vi "Double HWSync.vi"() -> ()   [LabVIEW 2014]
doc: "Use this template to build a producer/consumer design pattern with events to produce queue items. Use this design pattern instead of the User Interface Event Handler pattern for user interfaces when you want to execute code asynchronously in response to an event without slowing the user interface responsiveness."
uses:
  APIs/Message Queue/Enqueue Message (Single).vi
  APIs/Message Queue/Enqueue Message (Array).vi
  HWSyncLoop/HWSyncLoop.lvlib
  APIs/Message Queue/WINFAS 2 Message Queue.lvlib
panel:
  in  "SEND":bool
  in  "LOAD DRIVER":bool
  in  "Ruta a Driver":path=path "D:/Repositorio MAGNIS/INF002/v0/Modules/HAL/DriverMasterSync/build/DriverMasterSync.lvlibp"
  in  "Mensaje":string
  in  "stop":bool
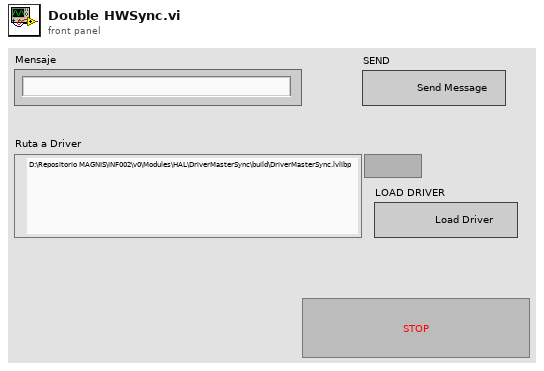
[diagram p1: front panel]
types:
  T1 = typedef "WINFAS 2 Message Queue.lvlib/All Message Queues.ctl" = cluster{"CORE":refnum<queue>, "HAL":refnum<queue>, "HWSync1":refnum<queue>, "HWSync2":refnum<queue>, "HWSync3":refnum<queue>, "HWSync4":refnum<queue>, "HWSync5":refnum<queue>, "HWAsync":refnum<queue>, "Event UI":refnum<queue>, "Display UI":refnum<queue>, "MATH":refnum<queue>, "SEQ":refnum<queue>, "DB":refnum<queue>, "ERR":refnum<queue>}
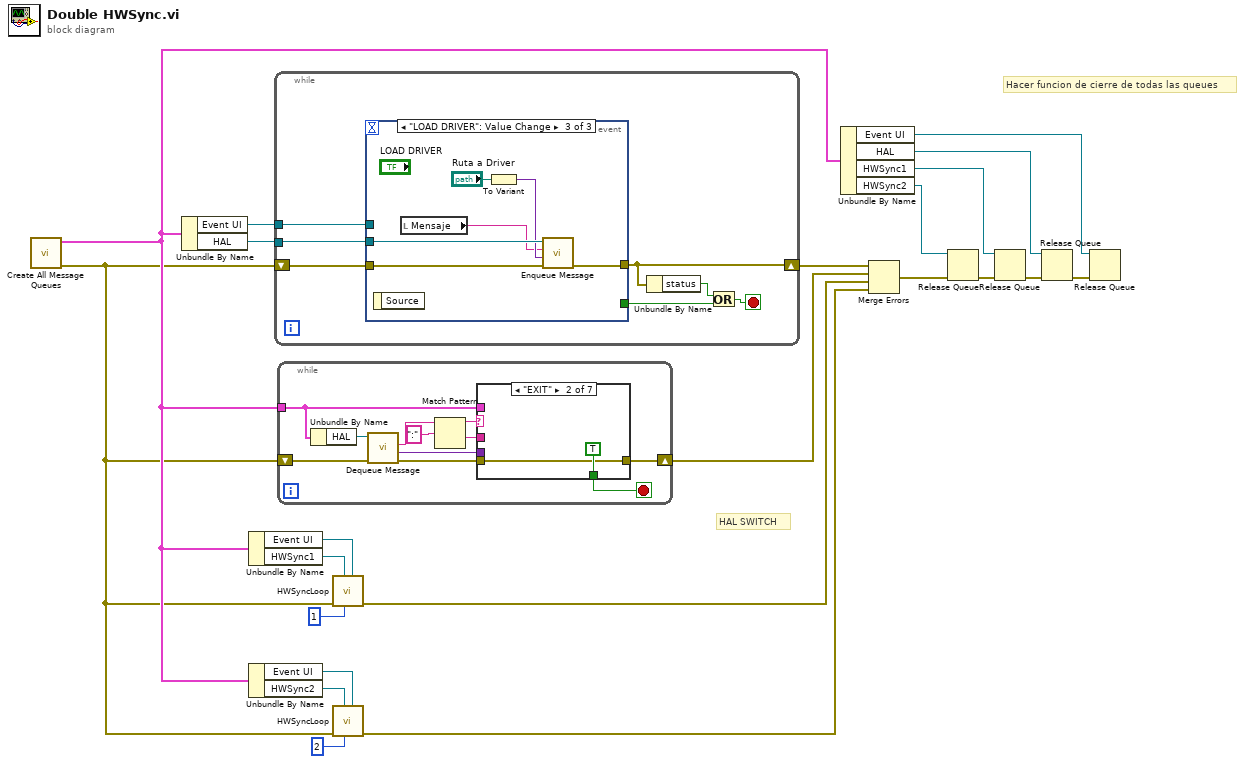
[diagram p0: block diagram]
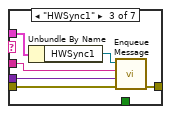
[diagram p3: hidden frame]
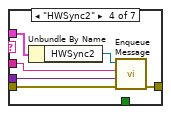
[diagram p4: hidden frame]
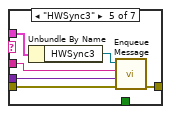
[diagram p5: hidden frame]
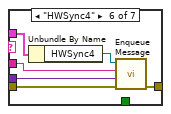
[diagram p6: hidden frame]
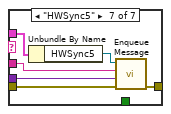
[diagram p7: hidden frame]
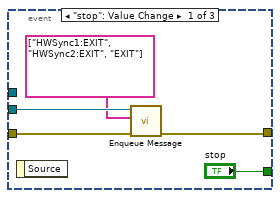
[diagram p8: hidden frame]
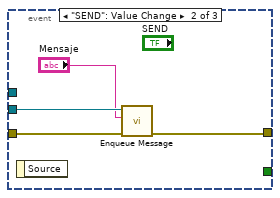
[diagram p9: hidden frame]
diagram:
  # "Hacer funcion de cierre de todas las queues"
  # "HAL SWITCH"
  n1 = call "Create All Message Queues.vi"() -> ("error out"=w4:errorcluster, "Message Queues out"=w6:T1)  [unwired: 10 in]
  n2 = Unbundle By Name(w6) -> ("Event UI"=w22:refnum<queue>, "HAL"=w17:refnum<queue>)
  n3 = Unbundle By Name(w6) -> ("Event UI"=w21:refnum<queue>, "HWSync1"=w20:refnum<queue>)
  n4 = Unbundle By Name(w6) -> ("Event UI"=w5:refnum<queue>, "HWSync2"=w7:refnum<queue>)
  n5 = while {
    shift-right: [w25] -> w18
    shift-left: w4 -> [w28]
    tunnel: w22 -> [w29]
    tunnel: w17 -> [w23]
    stop <- w26 stop-if-true
    n6 = event shown="[2] \"LOAD DRIVER\": Value Change" {
      selector: _ -> [_ _ _]
      dyn-events: _ -> [_ _ _]
      timeout: _ -> [_ _ _]
      tunnel: w29 -> [_ _ _]
      tunnel: w28 -> [w32 w38 w43]
      tunnel: [w31 w35 w41] -> w25
      tunnel: ["stop" _ _] -> w27
      tunnel: w23 -> [w33 w37 w42]
      event "stop": Value Change {
        n7 = event-data() -> ()  [unwired: 1 in, 1 out]
        n8 = call-poly "Enqueue Message.vi"("error in (no error)"=w32, "Message Array"=string[] ["HWSync1:EXIT", "HWSync2:EXIT", "EXIT"], "Message Queue"=w33) -> ("error out"=w31:errorcluster)  [unwired: 7 in, 1 out]
      }
      event "SEND": Value Change {
        n9 = event-data() -> ()  [unwired: 1 in, 1 out]
        n10 = call-poly "Enqueue Message.vi"("error in (no error)"=w38, "Message"="Mensaje", "Message Queue"=w37) -> ("error out"=w35:errorcluster)  [unwired: 7 in, 1 out]
      }
      event "LOAD DRIVER": Value Change {
        n11 = event-data() -> ()  [unwired: 1 in, 1 out]
        n12 = local read "Mensaje"() -> (w39:string)
        n13 = To Variant(anything="Ruta a Driver") -> (Variant=w40:variant)
        n14 = call-poly "Enqueue Message.vi"("error in (no error)"=w43, "Message Data"=w40, "Message"=w39, "Message Queue"=w42) -> ("error out"=w41:errorcluster)  [unwired: 6 in, 1 out]
      }
    }
    n15 = Unbundle By Name(w25) -> ("status"=w24:bool)
    n16 = Or(x=w24, y=w27) -> (x .or. y?=w26:bool)
  }
  n17 = while {
    tunnel: w6 -> [w49]
    shift-right: [w45] -> w15
    shift-left: w4 -> [w47]
    stop <- w48 stop-if-true
    n18 = Unbundle By Name(w49) -> ("HAL"=w55:refnum<queue>)
    n19 = call "Dequeue Message.vi"("error in (no error)"=w47, "Message Queue"=w55) -> ("error out"=w46:errorcluster, "Message Data"=w54:variant, "Message"=w53:string)  [unwired: 6 in, 1 out]
    n20 = Match Pattern(string=w53, regular expression=":") -> (before substring=w51:string, after substring=w50:string)  [unwired: 1 in, 2 out]
    n21 = case shown="\"EXIT\"" w51 {
      tunnel: w54 -> [_ _ w61 w67 w73 w79 w85]
      tunnel: w50 -> [_ _ w62 w68 w74 w80 w86]
      tunnel: w49 -> [_ _ w64 w70 w76 w82 w88]
      tunnel: [_ TRUE _ _ _ _ _] -> w48
      tunnel: w46 -> [w56 w57 w60 w66 w71 w77 w84]
      tunnel: [w56 w57 w59 w65 w72 w78 w83] -> w45
      frame Default {
      }
      frame "EXIT" {
      }
      frame "HWSync1" {
        n22 = Unbundle By Name(w64) -> ("HWSync1"=w63:refnum<queue>)
        n23 = call-poly "Enqueue Message.vi"("error in (no error)"=w60, "Message Data"=w61, "Message"=w62, "Message Queue"=w63) -> ("error out"=w59:errorcluster)  [unwired: 6 in, 1 out]
      }
      frame "HWSync2" {
        n24 = Unbundle By Name(w70) -> ("HWSync2"=w69:refnum<queue>)
        n25 = call-poly "Enqueue Message.vi"("error in (no error)"=w66, "Message Data"=w67, "Message"=w68, "Message Queue"=w69) -> ("error out"=w65:errorcluster)  [unwired: 6 in, 1 out]
      }
      frame "HWSync3" {
        n26 = Unbundle By Name(w76) -> ("HWSync3"=w75:refnum<queue>)
        n27 = call-poly "Enqueue Message.vi"("error in (no error)"=w71, "Message Data"=w73, "Message"=w74, "Message Queue"=w75) -> ("error out"=w72:errorcluster)  [unwired: 6 in, 1 out]
      }
      frame "HWSync4" {
        n28 = Unbundle By Name(w82) -> ("HWSync4"=w81:refnum<queue>)
        n29 = call-poly "Enqueue Message.vi"("error in (no error)"=w77, "Message Data"=w79, "Message"=w80, "Message Queue"=w81) -> ("error out"=w78:errorcluster)  [unwired: 6 in, 1 out]
      }
      frame "HWSync5" {
        n30 = Unbundle By Name(w88) -> ("HWSync5"=w87:refnum<queue>)
        n31 = call-poly "Enqueue Message.vi"("error in (no error)"=w84, "Message Data"=w85, "Message"=w86, "Message Queue"=w87) -> ("error out"=w83:errorcluster)  [unwired: 6 in, 1 out]
      }
    }
  }
  n32 = call "HWSyncLoop.vi"("CORE"=w21, "Num of Loop"=u8 1, "HWSync"=w20, "error in"=w4) -> ("error out"=w16:errorcluster)  [unwired: 7 in]
  n33 = call "HWSyncLoop.vi"("CORE"=w5, "Num of Loop"=u8 2, "HWSync"=w7, "error in"=w4) -> ("error out"=w3:errorcluster)  [unwired: 7 in]
  n34 = Unbundle By Name(w6) -> ("Event UI"=w11:refnum<queue>, "HAL"=w10:refnum<queue>, "HWSync1"=w9:refnum<queue>, "HWSync2"=w8:refnum<queue>)
  n35 = Merge Errors(w18, w15, w16, w3) -> (w13:errorcluster)
  n36 = Release Queue(queue=w8, error in (no error)=w13) -> (error out=w14:errorcluster)  [unwired: 1 in, 2 out]
  n37 = Release Queue(queue=w9, error in (no error)=w14) -> (error out=w12:errorcluster)  [unwired: 1 in, 2 out]
  n38 = Release Queue(queue=w10, error in (no error)=w12) -> (error out=w19:errorcluster)  [unwired: 1 in, 2 out]
  n39 = Release Queue(queue=w11, error in (no error)=w19) -> ()  [unwired: 1 in, 3 out]
